vi "Put One Chese.vi"(8 "column":i32, 9 "row":i32, 10 "current color":T2=2, 11 "data in":T1) -> (0 "available white position":i32[][](array[numeric]), 1 "available black position":i32[][](array[numeric]), 2 "new color":T2=2, 3 "data out":T1)   [LabVIEW 2018, in "Othello.xctl"]
doc: "本VI是为《我和LabVIEW》一书编写的示例。\n关于本书的介绍请参考网页：\nhttp://ruanqizhen.spaces.live.com/blog/cns!5852D4F797C53FB6!4310.entry"
uses:
  Othello.xctl
  Control/Pict Ring Chess.ctl
  Ability/Data.ctl
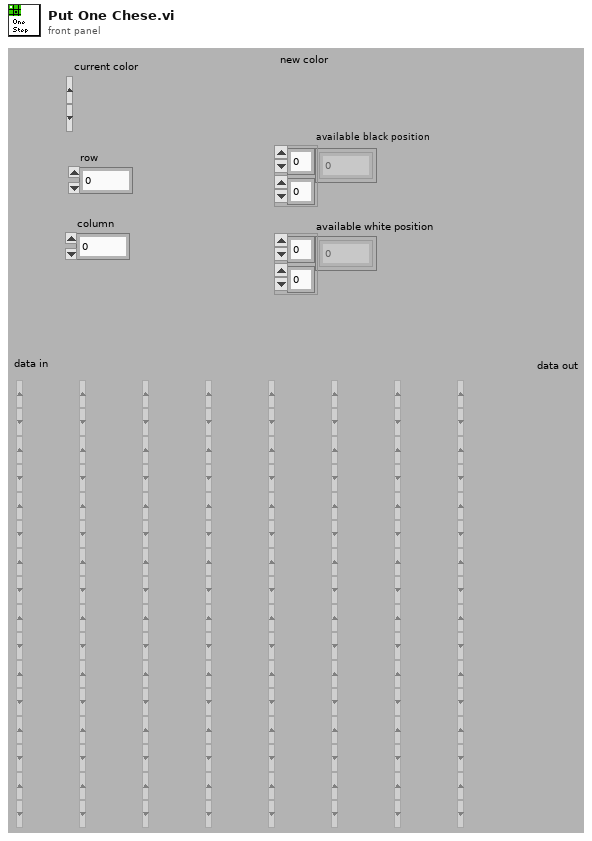
[diagram p1: front panel]
types:
  T1 = typedef "Othello.xctl/Data.ctl" = T2[][]
  T2 = typedef "Othello.xctl/Pict Ring Chess.ctl" = u16
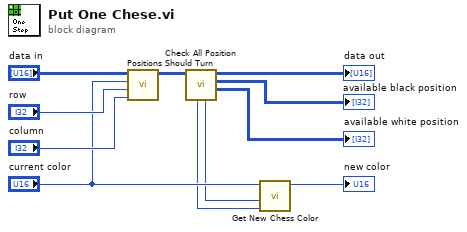
[diagram p0: block diagram]
diagram:
  n1 = call "Positions Should Turn.vi"("column"="column", "row"="row", "chess color"="current color", "chesses"="data in") -> ("chesses new"=w9:T1)  [unwired: 7 out]
  "data out" <- w9
  n2 = call "Check All Position.vi"("chesses"=w9) -> ("available white position"=→"available white position":i32[][], "available black position"=→"available black position":i32[][], "available black position number"=w2:i32, "available white position number"=w1:i32)  [unwired: 7 out]
  n3 = call "Get New Chess Color.vi"("white available position"=w1, "black available position"=w2, "current color"="current color") -> ("new color"=→"new color":T2)  [unwired: 3 in, 5 out]
